vi "NR_DePrecode.vi"(0 "appended path":path, 1 "TransformPrcode_en":dbl, 2 "prb_num":dbl, 3 "vnum":dbl, 4 "Nsym_slot":dbl, 5 "CodebookTransform_en":dbl, 6 "DMRS_symbol":dbl, 7 "TPMIindex":dbl, 9 "Antportnum":dbl, 11 "error in (no error)":errorcluster caption="错误输入（无错误）", 12 "equdata":cxt[](array[numeric])) -> (8 "delayermapdata":cdb[](array[numeric]), 15 "error IO":errorcluster)   [LabVIEW 2015]
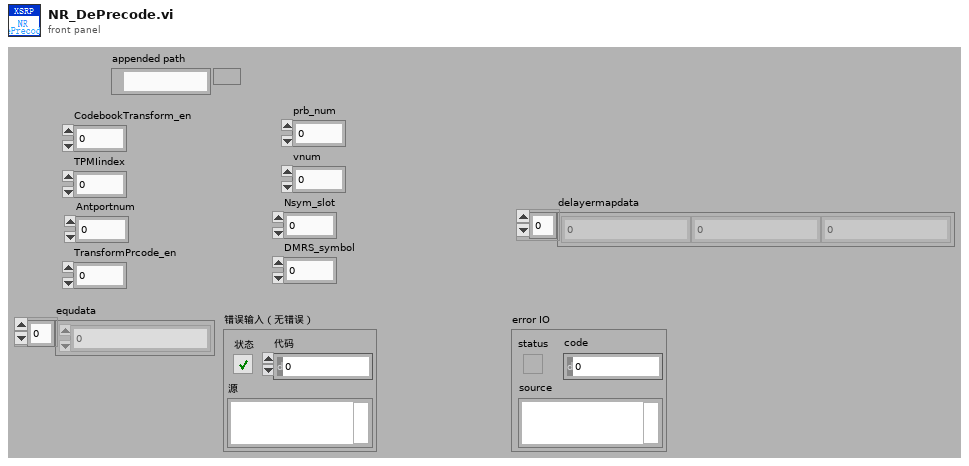
[diagram p1: front panel]
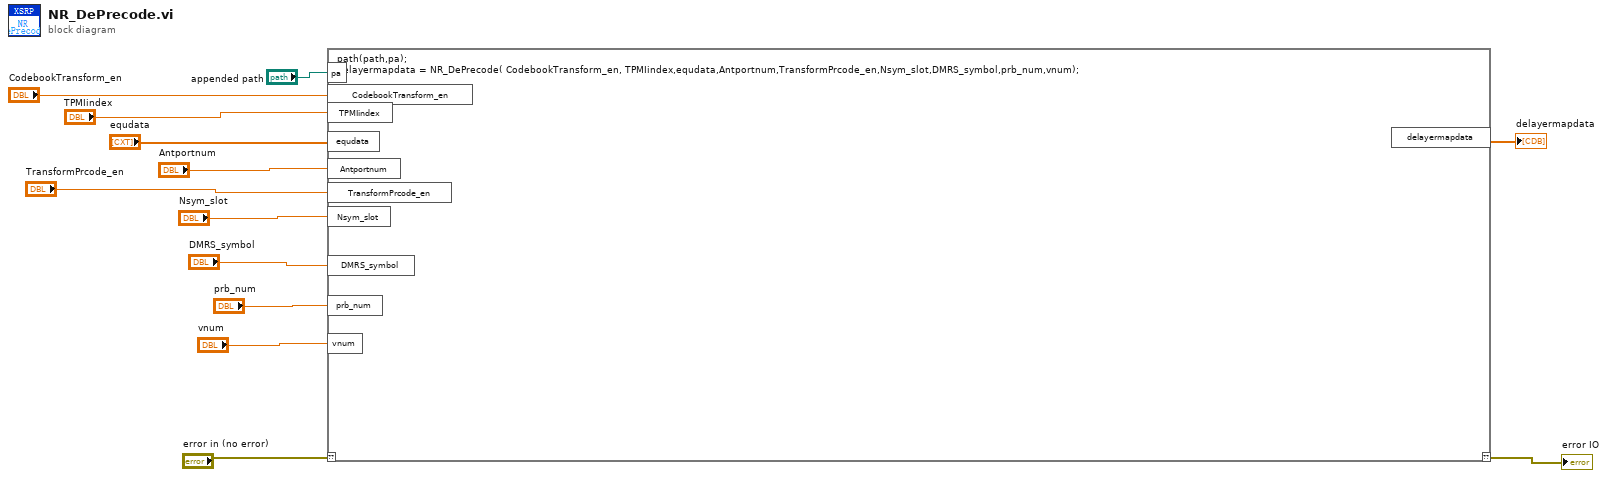
[diagram p0: block diagram]
diagram:
  n1 = script code="path(path,pa);\ndelayermapdata = NR_DePrecode( CodebookTransform_en, TPMIindex,equdata,Antportnum,TransformPrcode_en,Nsym_slot,DMRS_symbol,prb_num,vnum);"("??"="error in (no error)", "pa"="appended path", "CodebookTransform_en"="CodebookTransform_en", "TPMIindex"="TPMIindex", "equdata"="equdata", "Antportnum"="Antportnum", "TransformPrcode_en"="TransformPrcode_en", "Nsym_slot"="Nsym_slot", "DMRS_symbol"="DMRS_symbol", "prb_num"="prb_num", "vnum"="vnum") -> ("??"=→"error IO":errorcluster, "delayermapdata"=→"delayermapdata":cdb[])
